vi "KRM.vi"(0 "System no.":i32=1 min=1 max=4 step=1, 1 "Name":string, 5 "error in":errorcluster) -> (14 "Controller error":bool, 19 "error out":errorcluster)   [LabVIEW 2020]
doc: "Removes a coordinate system and queries ERR?. \nCoordinate system settings are volatile but can be saved as power-on default with WPA.vi using the password \"SKS\". If the coordinate system to remove is in use or does not exist, an error is set. If the coordinate system is used (e.g. part of an active chain), it cannot be removed.If a coordinate system which is part of a chain is removed, its parent and child are joined, so that the chain is still valid but KLT? results may differ. Coordinate systems of type KLD, KLF and KSB require command level 1 to remove them (CCL.vi). Controller error is TRUE if selected system reports error code not equal to 0. \n\nC-887, F-206, M-8X0: Only for GCS syntax version = GCS 2.0 or higher (Check with CSV?.vi. If CSV?.vi is not supported, syntax version is GCS 1.0)."
panel:
  # "Removes a coordinate system and queries ERR?."
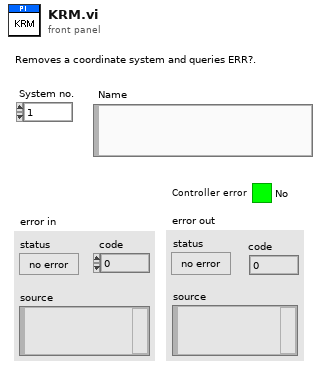
[diagram p1: front panel]
types:
  T1 = enum16{"Disable error check", "Force error check", "Use global settings"}
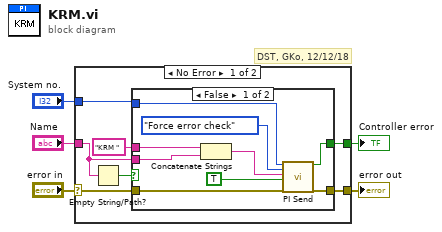
[diagram p0: block diagram]
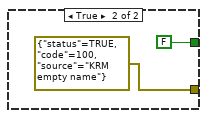
[diagram p2: hidden frame]
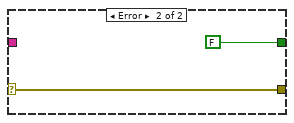
[diagram p3: hidden frame]
diagram:
  # "DST, GKo, 12/12/18"
  n1 = case shown="No Error" "error in" {
    selector: "error in" -> [w6 w24]
    tunnel: [w12 w24] -> w4
    tunnel: [w11 FALSE ("Controller error")] -> w5
    tunnel: "System no." -> [w10 _]
    tunnel: "Name" -> [w7 _]
    frame No Error {
      n2 = Empty String/Path?(string/path=w7) -> (empty?=w8:bool)
      n3 = case shown="False" w8 {
        tunnel: w6 -> [w21 _]
        tunnel: [w13 errorcluster {"status"=TRUE, "code"=100, "source"="KRM empty name"} ("error out")] -> w12
        tunnel: [w14 FALSE ("Controller error")] -> w11
        tunnel: w10 -> [w18 _]
        tunnel: "KRM " -> [w17 _]
        tunnel: w7 -> [w16 _]
        frame False {
          n4 = Concatenate Strings(w17, w16) -> (w19:string)
          n5 = call "PI Send.vi"("System no."=w18, "Error check settings"=T1."Force error check", "String to send"=w19, "Attach termination char.?"=TRUE ("Attach Linefeed?"), "error in"=w21) -> ("Controller error"=w14:bool, "error out"=w13:errorcluster)  [unwired: 1 in, 12 out]
        }
        frame True {
        }
      }
    }
    frame Error {
    }
  }
  "error out" <- w4
  "Controller error" <- w5
